vi "Digital Read 1 Channel.vi"(8 "error in (no error)":errorcluster, 10 "Read":i32, 11 "NI-DAQ in":refnum<class "NI-DAQ.lvclass">) -> (0 "error out":errorcluster, 2 "Value":bool=TRUE, 3 "NI-DAQ out":refnum<class "NI-DAQ.lvclass">)   [LabVIEW 2016, in "NI-DAQ.lvclass"]
uses:
  NI-DAQ.lvclass
panel:
  out "Boolean array":bool[](array[boolean])
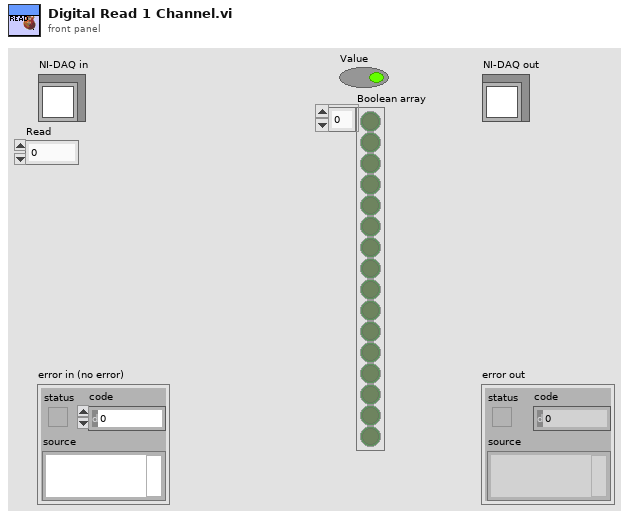
[diagram p1: front panel]
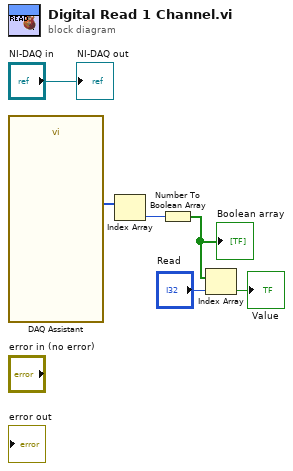
[diagram p0: block diagram]
diagram:
  n1 = call "DAQ Assistant"() -> ("data"=w6:u32[])  [unwired: 17 in, 2 out]
  n2 = Index Array(array=w6) -> (element=w5:u32)  [unwired: 1 in]
  n3 = Number To Boolean Array(number=w5) -> (Boolean array=w1:bool[])
  "Boolean array" <- w1
  n4 = Index Array(array=w1, index="Read") -> (element=→"Value":bool)
  "NI-DAQ out" <- "NI-DAQ in"
